vi "[GV]_STEER1.vi"() -> ()   [LabVIEW 2016]
panel:
  in  "STEER1":u16
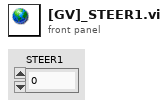
[diagram p1: front panel]
diagram:
